vi "Do.vi"(8 "error in (no error)":errorcluster, 10 "Actor in":refnum<class "Actor.lvclass">, 11 "Write ActorRefContainer Msg":refnum<class "Write ActorRefContainer Msg.lvclass">) -> (0 "error out":errorcluster, 2 "Actor out":refnum<class "Actor.lvclass">)   [LabVIEW 2019, in "ModuleAbstract.lvlib" / "Write ActorRefContainer Msg.lvclass"]
doc: "This VI delivers the message to the actor by calling the appropriate method(s) on the actor."
uses:
  Write ActorRefContainer Msg.lvclass
  <vilib>/ActorFramework/Actor/Actor.lvclass
  ModuleAbstract/ModuleAbstract.lvclass
  C:/Program Files (x86)/National Instruments/LabVIEW 2019/vi.lib/ActorFramework/Actor/Actor.lvclass
  Write ActorRefContainer Msg.lvclass/Write ActorRefContainer Msg.ctl
  ModuleAbstract/TypeDef/SelfQueue Msg.ctl
  ModuleAbstract/ModuleAbstract.lvclass/ModuleAbstract.ctl
  3efc70f7-1c3f-440c-a611-65722eff6af1.vi
  <vilib>/Utility/Data Type/Get Numeric Information.vi
  Containers/ActorRefContainer/ActorRefContainer.lvclass
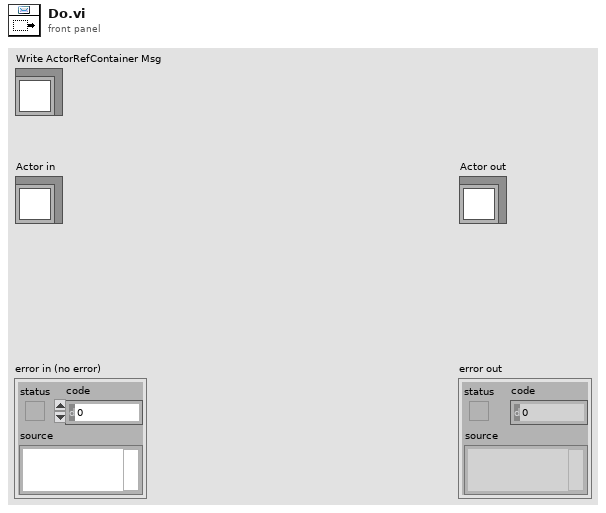
[diagram p1: front panel]
types:
  T1 = typedef "ModuleAbstract.lvlib/ModuleAbstract.lvclass/SelfQueue Msg.ctl" = enum16{"Read All Actors REF"}
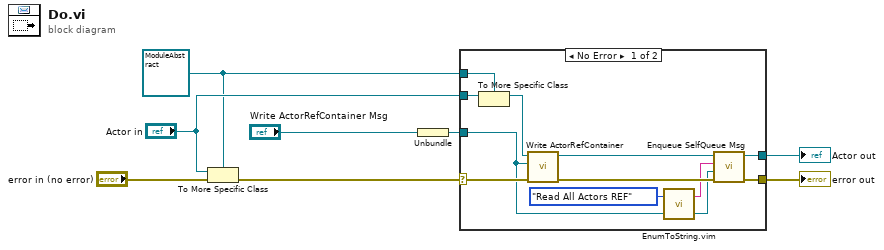
[diagram p0: block diagram]
diagram:
  w2 = refnum<class "ModuleAbstract.lvclass"> refnum ("Actor in")
  n1 = To More Specific Class(target class=w2, reference="Actor in", error in="error in (no error)") -> (error out=w6:errorcluster)  [unwired: 1 out]
  n2 = Unbundle("Write ActorRefContainer Msg") -> (w1:refnum<class "ActorRefContainer.lvclass">)
  n3 = case shown="No Error" w6 {
    selector: w6 -> [w19 w21]
    tunnel: [w11 w21] -> w5
    tunnel: [w12 w20] -> w4
    tunnel: "Actor in" -> [w18 w20]
    tunnel: w2 -> [w17 _]
    tunnel: w1 -> [w9 _]
    frame No Error {
      n4 = To More Specific Class(target class=w17, reference=w18) -> (specific class reference=w16:refnum<class "ModuleAbstract.lvclass">)  [unwired: 1 in, 1 out]
      n5 = call "Write ActorRefContainer.vi"("error in (no error)"=w19, "ActorRefContainer"=w9, "ModuleAbstract in"=w16) -> ("error out"=w13:errorcluster, "ModuleAbstract out"=w14:refnum<class "ModuleAbstract.lvclass">)  [unwired: 7 in]
      n6 = call "EnumToString.vim"("Enum"=SelfQueue_Msg."Read All Actors REF" ("SelfQueue Msg")) -> ("Enum Value"=w10:string)  [unwired: 16 in, 2 out]
      n7 = call "Enqueue SelfQueue Msg.vi"("error in (no error)"=w13, "Message Data"=w9, "Message"=w10, "ModuleAbstract in"=w14) -> ("error out"=w11:errorcluster, "ModuleAbstract out"=w12:refnum<class "ModuleAbstract.lvclass">)  [unwired: 6 in]
    }
    frame Error {
      # "If type check fails, pass the original object out again."
    }
  }
  "error out" <- w5
  "Actor out" <- w4
